vi "Order Patterns.vi"(8 "error in (no error)":errorcluster, 10 "Lithography Data":T2(array[cluster]), 11 "ListBox Reference in":refnum<vi>) -> (0 "error out":errorcluster, 1 "Order Unchanged":bool, 3 "Ordered Lithography Data":T2(array[cluster]))   [LabVIEW 2019]
uses:
  <userlib>/LevyLab/Relay Box/Typedefs/Resistor--enum.ctl
  <userlib>/LevyLab/Relay Box/Relay-Box.lvclass
panel:
  out "Order Litho Data":u32
  out "Get Names 2":u32
  out "Set Item Names":u32
  out "Get Names 1":u32
  out "Total":u32
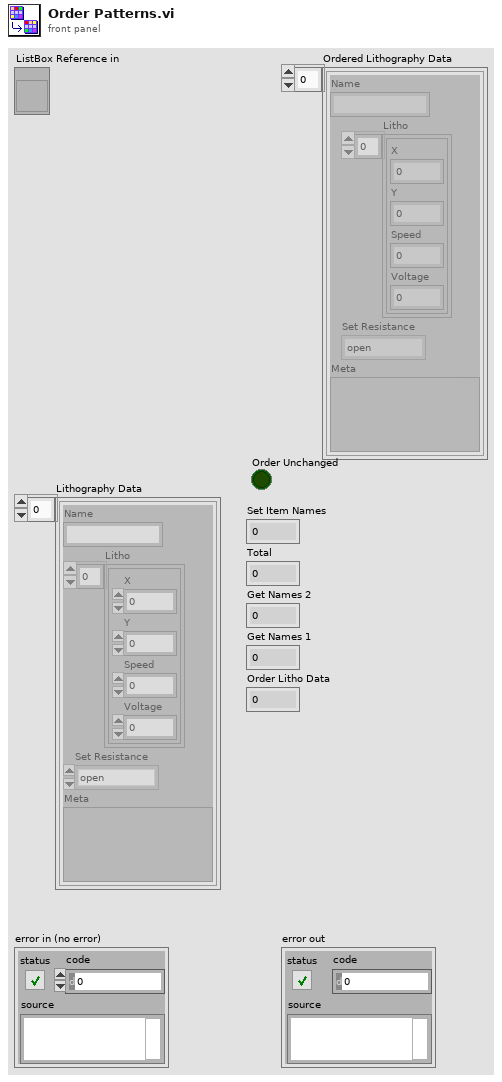
[diagram p1: front panel]
types:
  T1 = typedef "Relay-Box.lvclass/Resistor--enum.ctl" = enum16{"open", "discharge tip", "0 ohms", "100k ohm", "10M ohm", "1G ohm"}
  T2 = cluster{"Name":string, "Litho":cluster{"X":dbl, "Y":dbl, "Speed":dbl, "Voltage":dbl}[], "Set Resistance":T1, "Meta":variant}[]
  T3 = cluster{"Name":string, "Litho":cluster{"X":dbl, "Y":dbl, "Speed":dbl, "Voltage":dbl}[], "Set Resistance":T1, "Meta":variant}
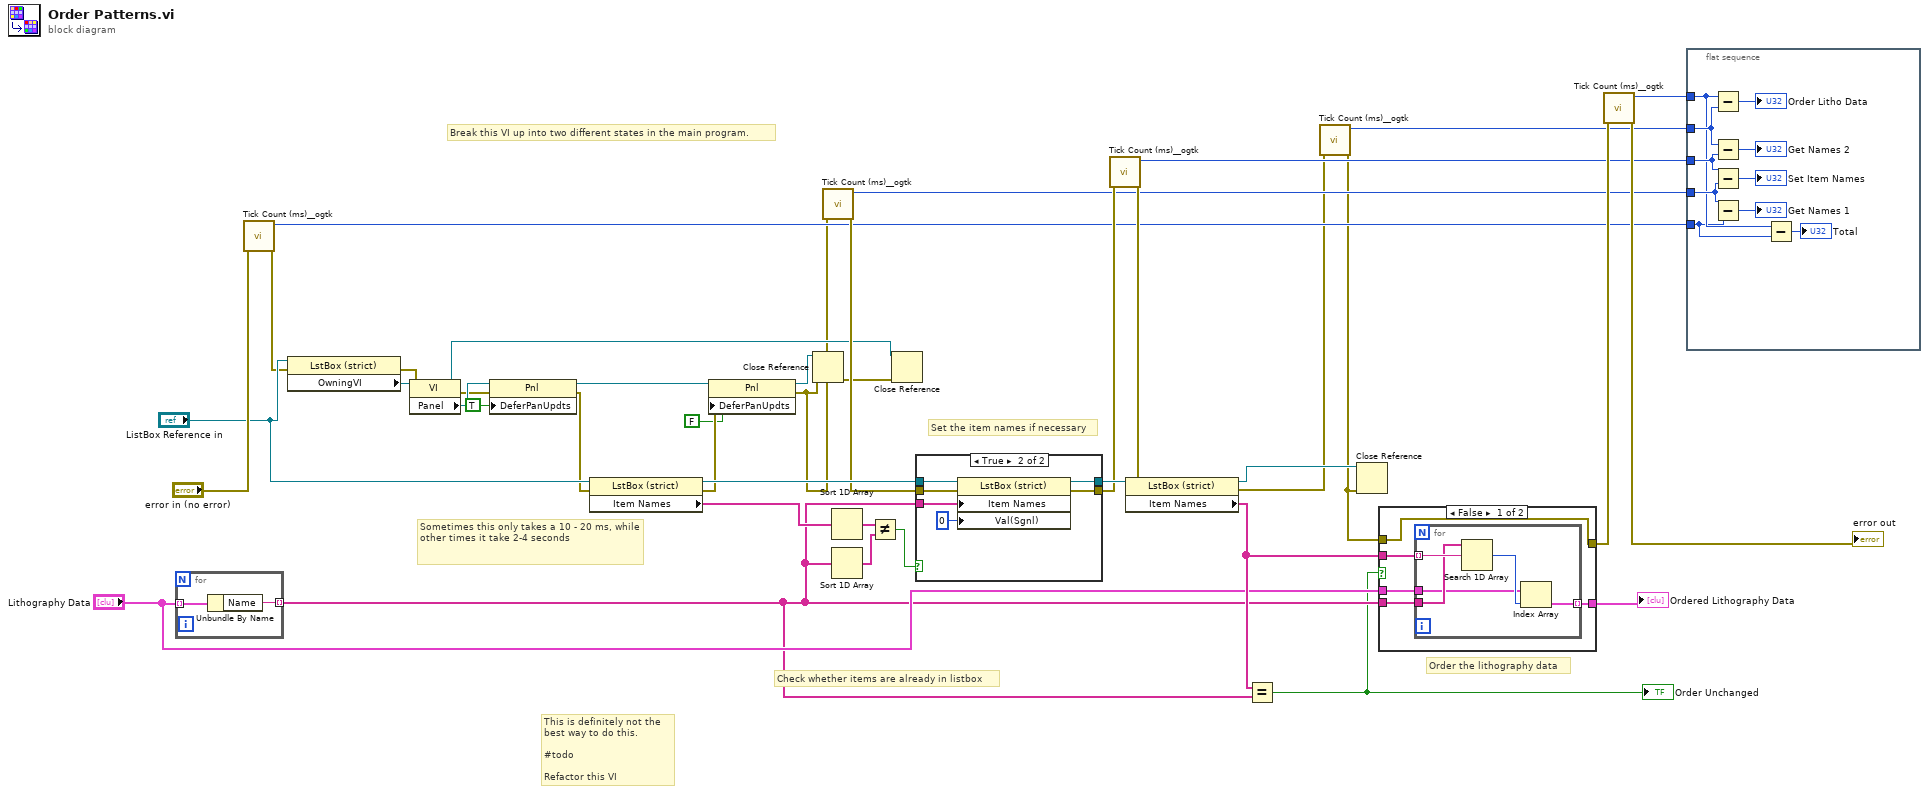
[diagram p0: block diagram]
diagram:
  # "Break this VI up into two different states in the main program."
  # "Sometimes this only takes a 10 - 20 ms, while other times it take 2-4 seconds"
  # "This is definitely not the best way to do this.\n\n#todo \n\nRefactor this VI"
  # "Check whether items are already in listbox"
  # "Set the item names if necessary"
  # "Order the lithography data"
  n1 = for {
    tunnel: "Lithography Data" -> [w42] mode=indexing
    tunnel: [w41] -> w30 mode=indexing
    n2 = Unbundle By Name(w42) -> ("Name"=w41:string)
  }
  n3 = call <userlib>:"Tick Count (ms)__ogtk.vi"("error in (no error)"="error in (no error)") -> ("error out"=w8:errorcluster, "millisecond timer value"=w18:u32)  [unwired: 9 in]
  n4 = property class="LstBox (strict)"(reference="ListBox Reference in", error in=w8) -> (error out=w10:errorcluster, "OwningVI"=w14:refnum<vi>)  [unwired: 1 out]
  n5 = property class="VI"(reference=w14, error in=w10) -> (reference out=w3:refnum<vi>, error out=w9:errorcluster, "Panel"=w13:refnum<vi>)
  n6 = property class="Pnl"(reference=w13, error in=w9, "DeferPanUpdts"=TRUE ("Defer Panel Updates")) -> (reference out=w6:refnum<vi>, error out=w11:errorcluster)
  n7 = property class="LstBox (strict)"(reference="ListBox Reference in", error in=w11) -> (reference out=w36:refnum<vi>, error out=w7:errorcluster, "Item Names"=w32:string[])
  n8 = property class="Pnl"(reference=w6, error in=w7, "DeferPanUpdts"=FALSE ("Defer Panel Updates")) -> (reference out=w4:refnum<vi>, error out=w2:errorcluster)
  n9 = Close Reference(reference=w4, error in (no error)=w2) -> (error out=w1:errorcluster)
  n10 = call <userlib>:"Tick Count (ms)__ogtk.vi"("error in (no error)"=w2) -> ("error out"=w26:errorcluster, "millisecond timer value"=w19:u32)  [unwired: 9 in]
  n11 = Sort 1D Array(array=w32) -> (sorted array=w37:string[])
  n12 = Sort 1D Array(array=w30) -> (sorted array=w38:string[])
  n13 = Not Equal?(x=w37, y=w38) -> (x != y?=w35:bool)
  n14 = Close Reference(reference=w3, error in (no error)=w1) -> ()  [unwired: 1 out]
  n15 = case shown="True" w35 {
    tunnel: w30 -> [_ w50]
    tunnel: w36 -> [w44 w49]
    tunnel: w26 -> [w43 w48]
    tunnel: [w43 w47] -> w24
    tunnel: [w44 w46] -> w40
    frame False {
    }
    frame True {
      n16 = property class="LstBox (strict)"(reference=w49, error in=w48, "Item Names"=w50, "Val(Sgnl)"=0 ("Value (Signaling)")) -> (reference out=w46:refnum<vi>, error out=w47:errorcluster)
    }
  }
  n17 = call <userlib>:"Tick Count (ms)__ogtk.vi"("error in (no error)"=w24) -> ("error out"=w23:errorcluster, "millisecond timer value"=w20:u32)  [unwired: 9 in]
  n18 = property class="LstBox (strict)"(reference=w40, error in=w23) -> (reference out=w39:refnum<vi>, error out=w16:errorcluster, "Item Names"=w33:string[])
  n19 = Equal?(x=w33, y=w30) -> (x = y?=w29:bool)
  "Order Unchanged" <- w29
  n20 = call <userlib>:"Tick Count (ms)__ogtk.vi"("error in (no error)"=w16) -> ("error out"=w17:errorcluster, "millisecond timer value"=w21:u32)  [unwired: 9 in]
  n21 = Close Reference(reference=w39, error in (no error)=w17) -> ()  [unwired: 1 out]
  n22 = case shown="False" w29 {
    tunnel: [w55 w62] -> w34
    tunnel: w33 -> [w54 _]
    tunnel: "Lithography Data" -> [w53 w62]
    tunnel: w30 -> [w52 _]
    tunnel: w17 -> [w51 w61]
    tunnel: [w51 w61] -> w27
    frame False {
      n23 = for {
        tunnel: w54 -> [w60] mode=indexing
        tunnel: w52 -> [w58]
        tunnel: [w57] -> w55 mode=indexing
        tunnel: w53 -> [w56]
        n24 = Search 1D Array(1D array=w58, element=w60) -> (index of element=w59:i32)  [unwired: 1 in]
        n25 = Index Array(array=w56, index=w59) -> (element=w57:T3)
      }
    }
    frame True {
    }
  }
  "Ordered Lithography Data" <- w34
  n26 = call <userlib>:"Tick Count (ms)__ogtk.vi"("error in (no error)"=w27) -> ("error out"=→"error out":errorcluster, "millisecond timer value"=w22:u32)  [unwired: 9 in]
  n27 = flat-sequence {
    tunnel: w22 -> [w69]
    tunnel: w21 -> [w72]
    tunnel: w20 -> [w71]
    tunnel: w19 -> [w70]
    tunnel: w18 -> [w63]
    frame #0 {
      n28 = Subtract(x=w69, y=w72) -> (x-y=→"Order Litho Data":u32)
      n29 = Subtract(x=w72, y=w71) -> (x-y=→"Get Names 2":u32)
      n30 = Subtract(x=w71, y=w70) -> (x-y=→"Set Item Names":u32)
      n31 = Subtract(x=w70, y=w63) -> (x-y=→"Get Names 1":u32)
      n32 = Subtract(x=w69, y=w63) -> (x-y=→"Total":u32)
    }
  }
